vi "Check Empty in new case.vi"(11 "New Case":refnum<vi>) -> (3 "No Empty fields":bool)   [LabVIEW 2015]
uses:
  controls/Add New Case.ctl
  controls/Program.ctl
  controls/Type.ctl
  controls/Case Status.ctl
  controls/Date.ctl
  controls/Declined.ctl
  controls/Back to Business.ctl
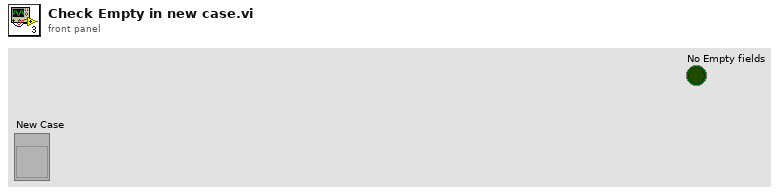
[diagram p1: front panel]
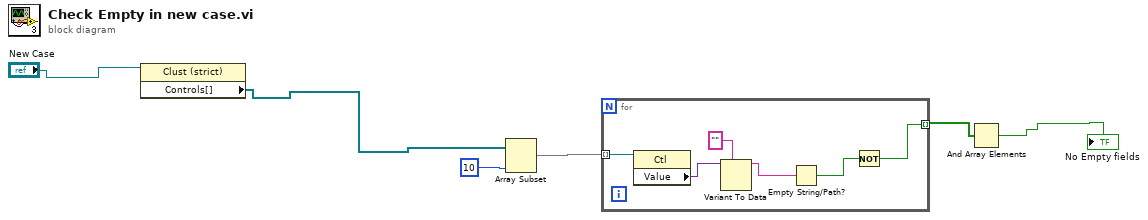
[diagram p0: block diagram]
diagram:
  n1 = property class="Clust (strict)"(reference="New Case") -> ("Controls[]"=w4:refnum<vi>[])  [unwired: 1 in, 2 out]
  n2 = Array Subset(array=w4, length=10) -> (w6:refnum<vi>[])  [unwired: 1 in]
  n3 = for {
    tunnel: w6 -> [w12] mode=indexing
    tunnel: [w10] -> w3 mode=indexing
    n4 = property class="Ctl"(reference=w12) -> ("Value"=w9:variant)  [unwired: 1 in, 2 out]
    n5 = Variant To Data(type="", Variant=w9) -> (data=w7:string)  [unwired: 1 in, 1 out]
    n6 = Empty String/Path?(string/path=w7) -> (empty?=w11:bool)
    n7 = Not(x=w11) -> (.not. x?=w10:bool)
  }
  n8 = And Array Elements(Boolean array=w3) -> (logical AND=→"No Empty fields":bool)
